vi "Field Scouting.vi"() -> ()   [LabVIEW 2015]
uses:
  <vilib>/Utility/sysdir.llb/System Directory Type.ctl
panel:
  in  "Comments":string
  in  "Low Goals Auto":dbl format="%#_4g"
  in  "High Goals Auto":dbl format="%#_4g"
  in  "?":bool
  in  "Rating":dbl=1.0 min=1.0 max=10.0 step=1.0
  in  "Low Goals":dbl format="%#_4g"
  in  "High Goals":dbl format="%#_4g"
  in  "Team Number":dbl format="%#_4g"
  in  "Scale?":bool
  in  "Auto?":bool
  in  "Tele Pass 5":bool
  in  "Tele Pass 4":bool
  in  "Tele Pass 3":bool
  in  "Tele Pass 2":bool
  in  "Tele Pass 1":bool
  in  "Auto Def 4":bool
  in  "Auto Def 3":bool
  in  "Auto Def 2":bool
  in  "Auto Def 1":bool
  in  "Touch 1":bool
  in  "Pass 5":bool
  in  "Pass 4":bool
  in  "Pass 3":bool
  in  "Pass 2":bool
  in  "Pass 1":bool
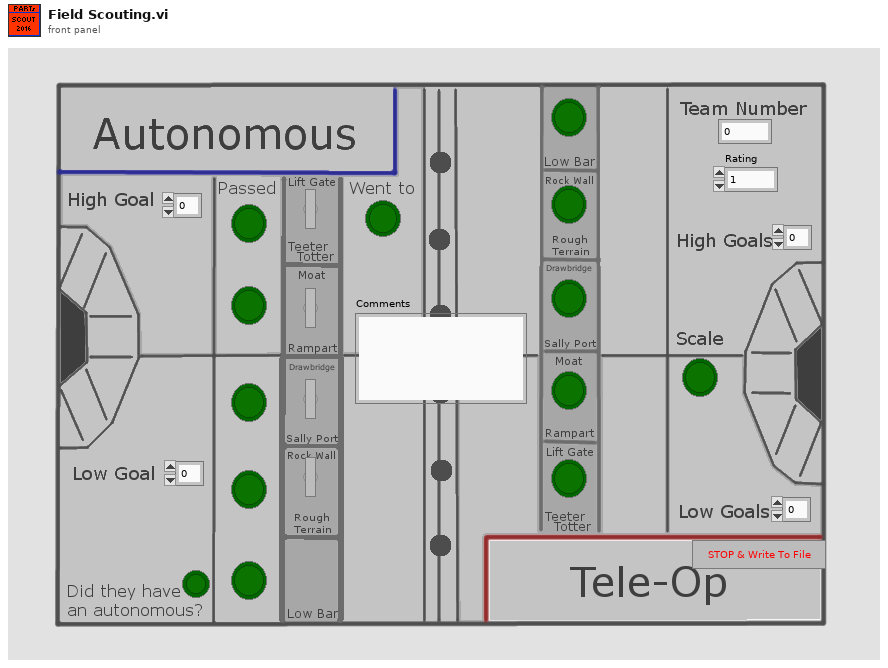
[diagram p1: front panel]
types:
  T1 = typedef "System Directory Type.ctl" = i32
  T2 = enum16{"open", "replace", "create", "open or create", "replace or create", "replace or create with confirmation"}
  T3 = enum32{"invalid app kind", "Development System", "Run Time System", "Student Edition", "Embedded LabVIEW", "Evaluation", "Custom"}
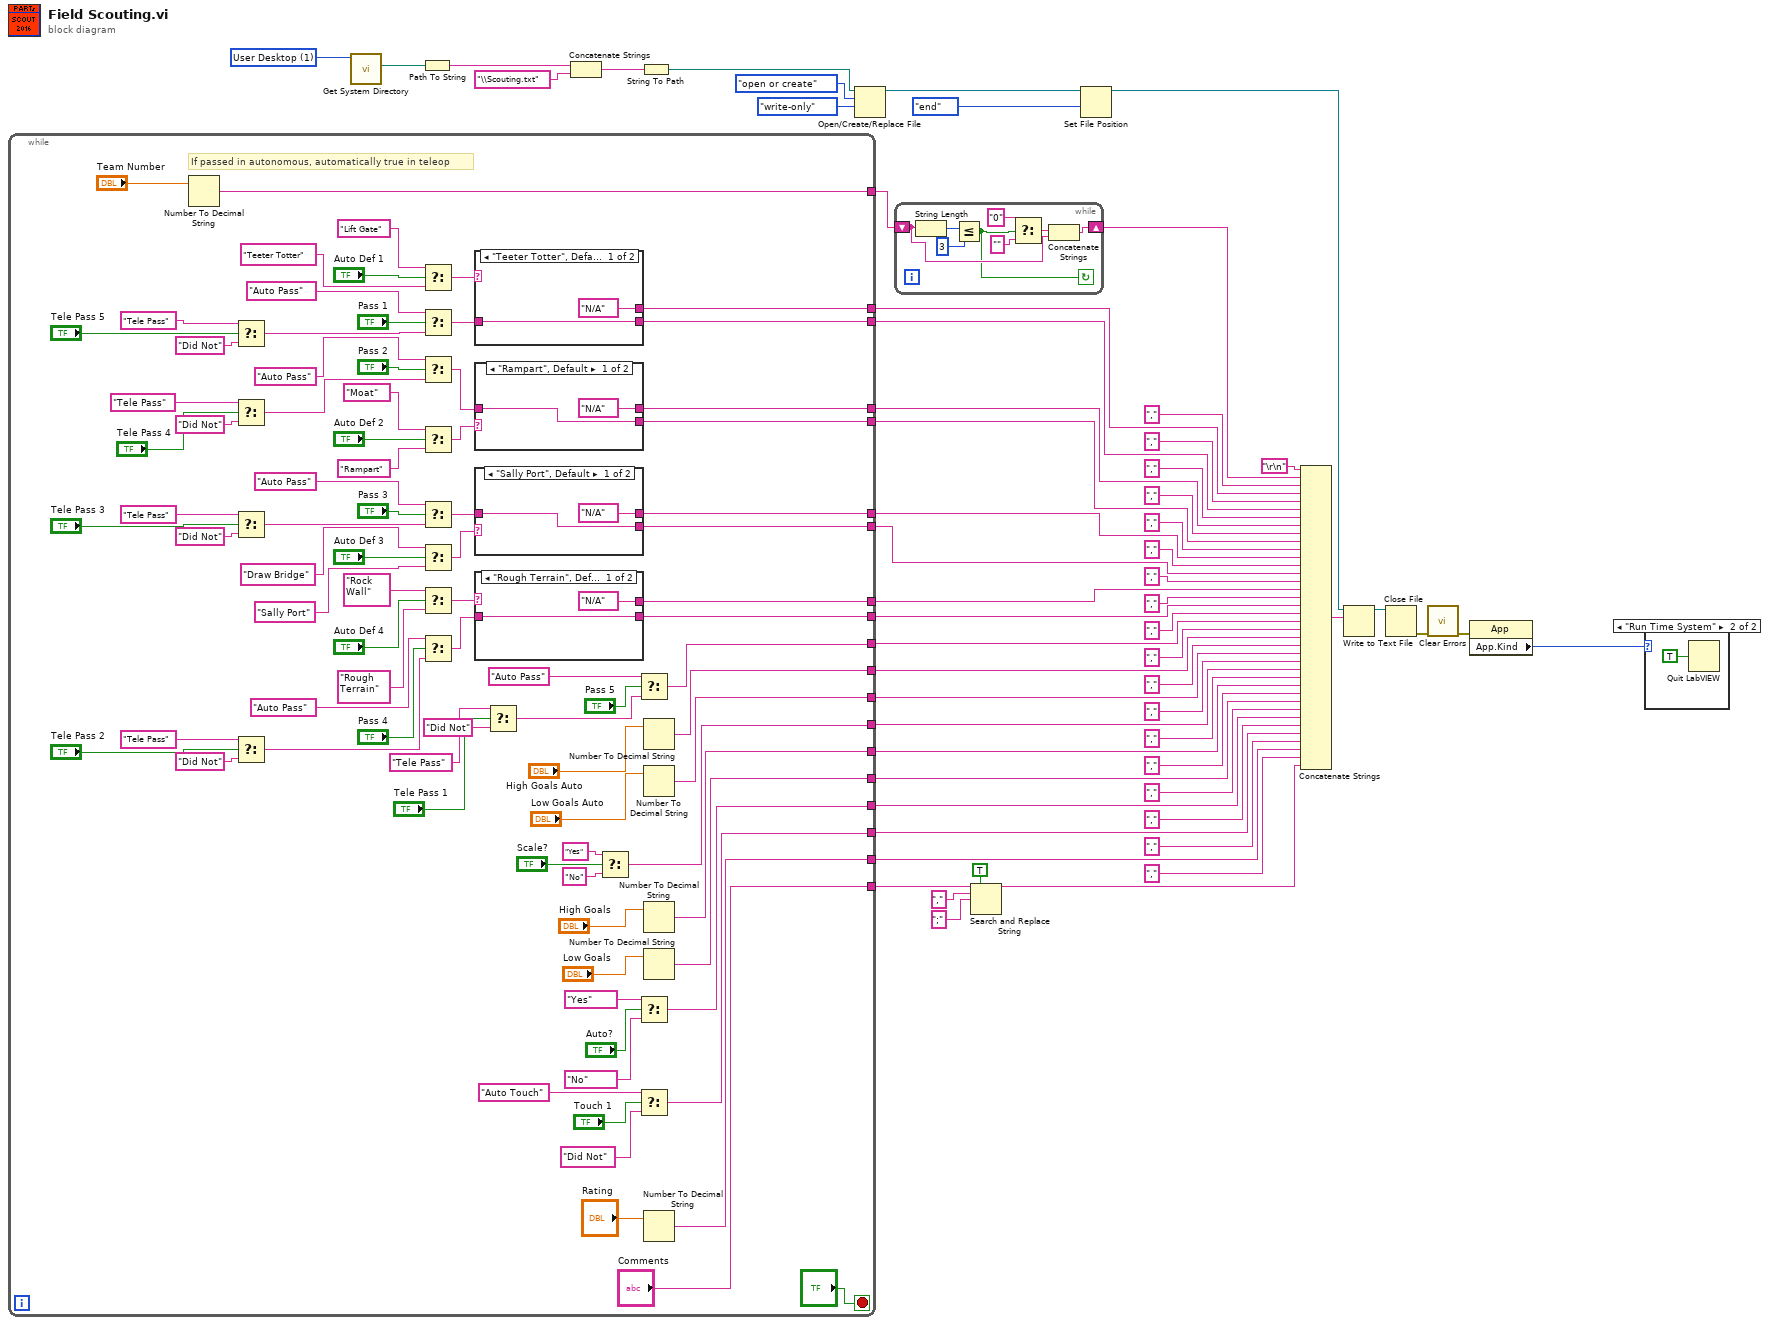
[diagram p0: block diagram]
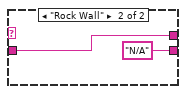
[diagram p2: hidden frame]
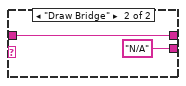
[diagram p3: hidden frame]
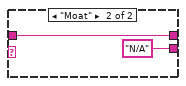
[diagram p4: hidden frame]
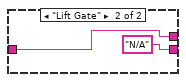
[diagram p5: hidden frame]
diagram:
  w22 = T1 1 items=["User Home"=0, "User Desktop"=1, "User Documents"=2, "User Application Data"=3, "User Preferences"=4, "User Temporary"=5, "Public Documents"=6, "Public Application Data"=7, "Public Preferences"=8, "Public Cache"=13, "System Core Libraries"=9, "System Installed Libraries"=10, "Application Files"=11, "Boot Volume Root"=12] ("system directory type")
  n1 = while {
    tunnel: [w60] -> w7
    tunnel: [w86] -> w46
    tunnel: [w85] -> w45
    tunnel: [w84] -> w44
    tunnel: [w83] -> w43
    tunnel: [w82] -> w42
    tunnel: [w81] -> w41
    tunnel: [w80] -> w40
    tunnel: [w79] -> w39
    tunnel: [w78] -> w38
    tunnel: [w64] -> w37
    tunnel: [w62] -> w33
    tunnel: [w77] -> w32
    tunnel: [w76] -> w31
    tunnel: [w75] -> w30
    tunnel: [w74] -> w29
    tunnel: [w72] -> w10
    tunnel: [w66] -> w12
    tunnel: ["Comments"] -> w4
    stop <- "?" stop-if-true
    # "If passed in autonomous, automatically true in teleop"
    n2 = Number To Decimal String(number="Team Number") -> (decimal integer string=w60:string)  [unwired: 1 in]
    n3 = Select(t="Tele Pass", s="Tele Pass 5", f="Did Not") -> (s? t:f=w100:string)
    n4 = Select(t="Tele Pass", s="Tele Pass 4", f="Did Not") -> (s? t:f=w98:string)
    n5 = Select(t="Tele Pass", s="Tele Pass 3", f="Did Not") -> (s? t:f=w94:string)
    n6 = Select(t="Tele Pass", s="Tele Pass 2", f="Did Not") -> (s? t:f=w91:string)
    n7 = Select(t="Lift Gate", s="Auto Def 1", f="Teeter Totter") -> (s? t:f=w108:string)
    n8 = Select(t="Auto Pass", s="Pass 1", f=w100) -> (s? t:f=w99:string)
    n9 = Select(t="Auto Pass", s="Pass 2", f=w98) -> (s? t:f=w97:string)
    n10 = Select(t="Moat", s="Auto Def 2", f="Rampart") -> (s? t:f=w96:string)
    n11 = Select(t="Auto Pass", s="Pass 3", f=w94) -> (s? t:f=w92:string)
    n12 = Select(t="Draw Bridge", s="Auto Def 3", f="Sally Port") -> (s? t:f=w93:string)
    n13 = Select(t="Rock Wall", s="Auto Def 4", f="Rough Terrain") -> (s? t:f=w89:string)
    n14 = Select(t="Auto Pass", s="Pass 4", f=w91) -> (s? t:f=w90:string)
    n15 = case shown="\"Teeter Totter\", Default" w108 {
      tunnel: [w158 "N/A" ("t")] -> w85
      tunnel: w99 -> [w158 w160]
      tunnel: ["N/A" w160] -> w86
      frame "Teeter Totter", Default {
      }
      frame "Lift Gate" {
      }
    }
    n16 = case shown="\"Rampart\", Default" w96 {
      tunnel: [w154 "N/A" ("t")] -> w83
      tunnel: w97 -> [w154 w156]
      tunnel: ["N/A" w156] -> w84
      frame "Rampart", Default {
      }
      frame "Moat" {
      }
    }
    n17 = case shown="\"Sally Port\", Default" w93 {
      tunnel: [w150 "N/A" ("t")] -> w81
      tunnel: w92 -> [w150 w152]
      tunnel: ["N/A" w152] -> w82
      frame "Sally Port", Default {
      }
      frame "Draw Bridge" {
      }
    }
    n18 = case shown="\"Rough Terrain\", Default" w89 {
      tunnel: [w146 "N/A" ("t")] -> w79
      tunnel: w90 -> [w146 w148]
      tunnel: ["N/A" w148] -> w80
      frame "Rough Terrain", Default {
      }
      frame "Rock Wall" {
      }
    }
    n19 = Select(t="Tele Pass", s="Tele Pass 1", f="Did Not") -> (s? t:f=w87:string)
    n20 = Select(t="Yes", s="Scale?", f="No") -> (s? t:f=w77:string)
    n21 = Select(t="Auto Pass", s="Pass 5", f=w87) -> (s? t:f=w78:string)
    n22 = Select(t="Yes", s="Auto?", f="No") -> (s? t:f=w74:string)
    n23 = Select(t="Auto Touch", s="Touch 1", f="Did Not") -> (s? t:f=w66:string)
    n24 = Number To Decimal String(number="High Goals Auto") -> (decimal integer string=w64:string)  [unwired: 1 in]
    n25 = Number To Decimal String(number="Low Goals Auto") -> (decimal integer string=w62:string)  [unwired: 1 in]
    n26 = Number To Decimal String(number="High Goals") -> (decimal integer string=w76:string)  [unwired: 1 in]
    n27 = Number To Decimal String(number="Low Goals") -> (decimal integer string=w75:string)  [unwired: 1 in]
    n28 = Number To Decimal String(number="Rating") -> (decimal integer string=w72:string)  [unwired: 1 in]
  }
  n29 = call <vilib>:"Get System Directory.vi"("system directory type"=w22) -> ("system directory"=w21:path)  [unwired: 10 in]
  n30 = Path To String(path=w21) -> (string=w20:string)
  n31 = Concatenate Strings(w20, "\\Scouting.txt" ("string")) -> (w18:string)
  n32 = String To Path(string=w18) -> (path=w17:path)
  n33 = Open/Create/Replace File(file path (use dialog)=w17, operation (0:open)=T2."open or create", access (0:read/write)=enum16{"read/write", "read-only", "write-only"}."write-only") -> (refnum out=w25:refnum<file>)  [unwired: 3 in, 2 out]
  n34 = while {
    shift-right: [w163] -> w6
    shift-left: w7 -> [w162]
    stop <- w161 continue-if-true
    n35 = String Length(string=w162) -> (length=w167:i32)
    n36 = Less Or Equal?(x=w167, y=3) -> (x <= y?=w161:bool)
    n37 = Select(t="0" ("string"), s=w161, f="") -> (s? t:f=w165:string)
    n38 = Concatenate Strings(w165, w162) -> (w163:string)
  }
  n39 = Search and Replace String(replace all?=TRUE ("replace all? (F)"), input string=w4, search string=",", replace string=";" ("replace string (\"\")")) -> (result string=w3:string)  [unwired: 4 in, 3 out]
  n40 = Set File Position(refnum=w25, from (0:start)=enum16{"start", "end", "current"}."end") -> (refnum out=w24:refnum<file>)  [unwired: 2 in, 1 out]
  n41 = Concatenate Strings("\r\n", w6, "," ("string"), w46, "," ("string"), w45, "," ("string"), w44, "," ("string"), w43, "," ("string"), w42, "," ("string"), w41, "," ("string"), w40, "," ("string"), w39, "," ("string"), w38, "," ("string"), w37, "," ("string"), w33, "," ("string"), w32, "," ("string"), w31, "," ("string"), w30, "," ("string"), w29, "," ("string"), w12, "," ("string"), w10, "," ("string"), w3) -> (w13:string)
  n42 = Write to Text File(file (use dialog)=w24, text=w13) -> (refnum out=w26:refnum<file>)  [unwired: 2 in, 2 out]
  n43 = Close File(refnum=w26) -> (error out=w16:errorcluster)  [unwired: 1 in, 1 out]
  n44 = call <vilib>:"Clear Errors.vi"("error in (no error)"=w16) -> ("error out"=w15:errorcluster)  [unwired: 5 in, 1 out]
  n45 = property class="App"(error in=w15) -> ("App.Kind"=w14:T3)  [unwired: 1 in, 2 out]
  n46 = case shown="\"Run Time System\"" w14 {
    frame Default {
    }
    frame "Run Time System" {
      n47 = Quit LabVIEW(quit? (T)=TRUE) -> ()
    }
  }
